vi "RTS Sequence Logic.vi"(4 "Relay Number":u8=1 min=1 max=3 step=1, 5 "Delay":bool, 6 "Current Status":string[](array[string]), 7 "Station 1-8 Data in":T2 {"Station Slide"."Chamber 1-1"."Start Time" format="%<%X\n%x>T"; "Station Slide"."Chamber 1-1"."End Time" format="%<%X\n%x>T"; "Station Slide"."Time Count (s)" format="%.2f"; "Station Cab"."Chamber 1-1"."Start Time" format="%<%X\n%x>T"; "Station Cab"."Chamber 1-1"."End Time" format="%<%X\n%x>T"; "Station Cab"."Time Count (s)" format="%.2f"; "Station Freezer"."Chamber 1-1"."Start Time" format="%<%X\n%x>T"; "Station Freezer"."Chamber 1-1"."End Time" format="%<%X\n%x>T"; "Station Freezer"."Time Count (s)" format="%.2f"}, 8 "error in (no error)":errorcluster, 10 "Door Open Delay(sec)":dbl, 11 "Door Open Sequence:":T1) -> (0 "error out":errorcluster, 2 "Run Door Op Sequence":bool, 3 "Station 1-8 Data out":T2 {"Station Slide"."Chamber 1-1"."Start Time" format="%<%X\n%x>T"; "Station Slide"."Chamber 1-1"."End Time" format="%<%X\n%x>T"; "Station Slide"."Time Count (s)" format="%.2f"; "Station Cab"."Chamber 1-1"."Start Time" format="%<%X\n%x>T"; "Station Cab"."Chamber 1-1"."End Time" format="%<%X\n%x>T"; "Station Cab"."Time Count (s)" format="%.2f"; "Station Freezer"."Chamber 1-1"."Start Time" format="%<%X\n%x>T"; "Station Freezer"."Chamber 1-1"."End Time" format="%<%X\n%x>T"; "Station Freezer"."Time Count (s)" format="%.2f"})   [LabVIEW 2016]
uses:
  Type Definitions/RTS Station Relay Ops.ctl
  Type Definitions/RTS Door Opener Indicator.ctl
  Type Definitions/RTS Door Ops Client.ctl
  Type Definitions/RTS Door Opening Schedule.ctl
  Type Definitions/RTS Door Ops Sequence.ctl
panel:
  # "Chamber Conditions:"
  # "Chamber Conditions:"
  # "Chamber Conditions:"
  # "Chamber Conditions:"
  # "Chamber Conditions:"
  # "Chamber Conditions:"
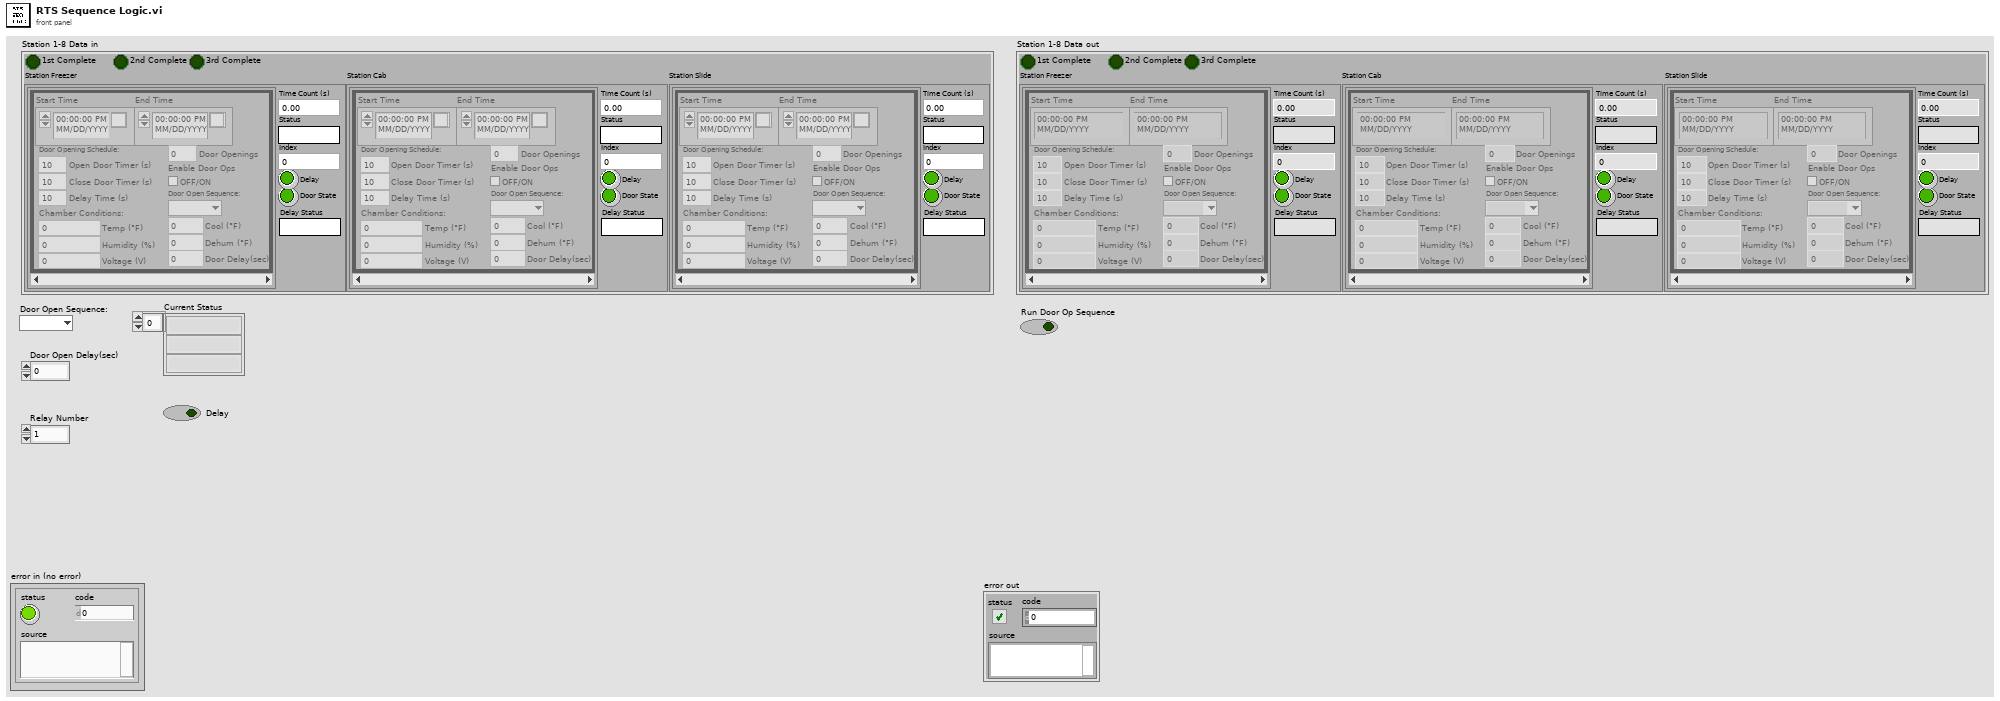
[diagram p1: front panel]
types:
  T1 = typedef "RTS Door Ops Sequence.ctl" = enum16{"", "1st", "2nd", "3rd"}
  T2 = typedef "RTS Station Relay Ops.ctl" = cluster{"Station Freezer":T3, "Station Cab":T3, "Station Slide":T3, "1st Complete":bool, "2nd Complete":bool, "3rd Complete":bool}
  T3 = typedef "RTS Door Opener Indicator.ctl" = cluster{"Time Count (s)":dbl, "Status":string, "Door State":bool, "Delay":bool, "Chamber 1-1":T4[], "Index":i32, "Delay Status":string}
  T4 = typedef "RTS Door Ops Client.ctl" = cluster{"End Time":timestamp, "Start Time":timestamp, "Door Opening Schedule:":T5, "Enable Door Ops":bool, "Door Openings":u32, "Temp (°F)":dbl, "Humidity (%)":dbl, "Voltage (V)":dbl, "Door Open Sequence:":T1, "Door Delay(sec)":dbl, "Dehum (°F)":dbl, "Cool (°F)":dbl}
  T5 = typedef "RTS Door Opening Schedule.ctl" = cluster{"Open Door Timer (s)":dbl, "Delay Time (s)":dbl, "Close Door Timer (s)":dbl}
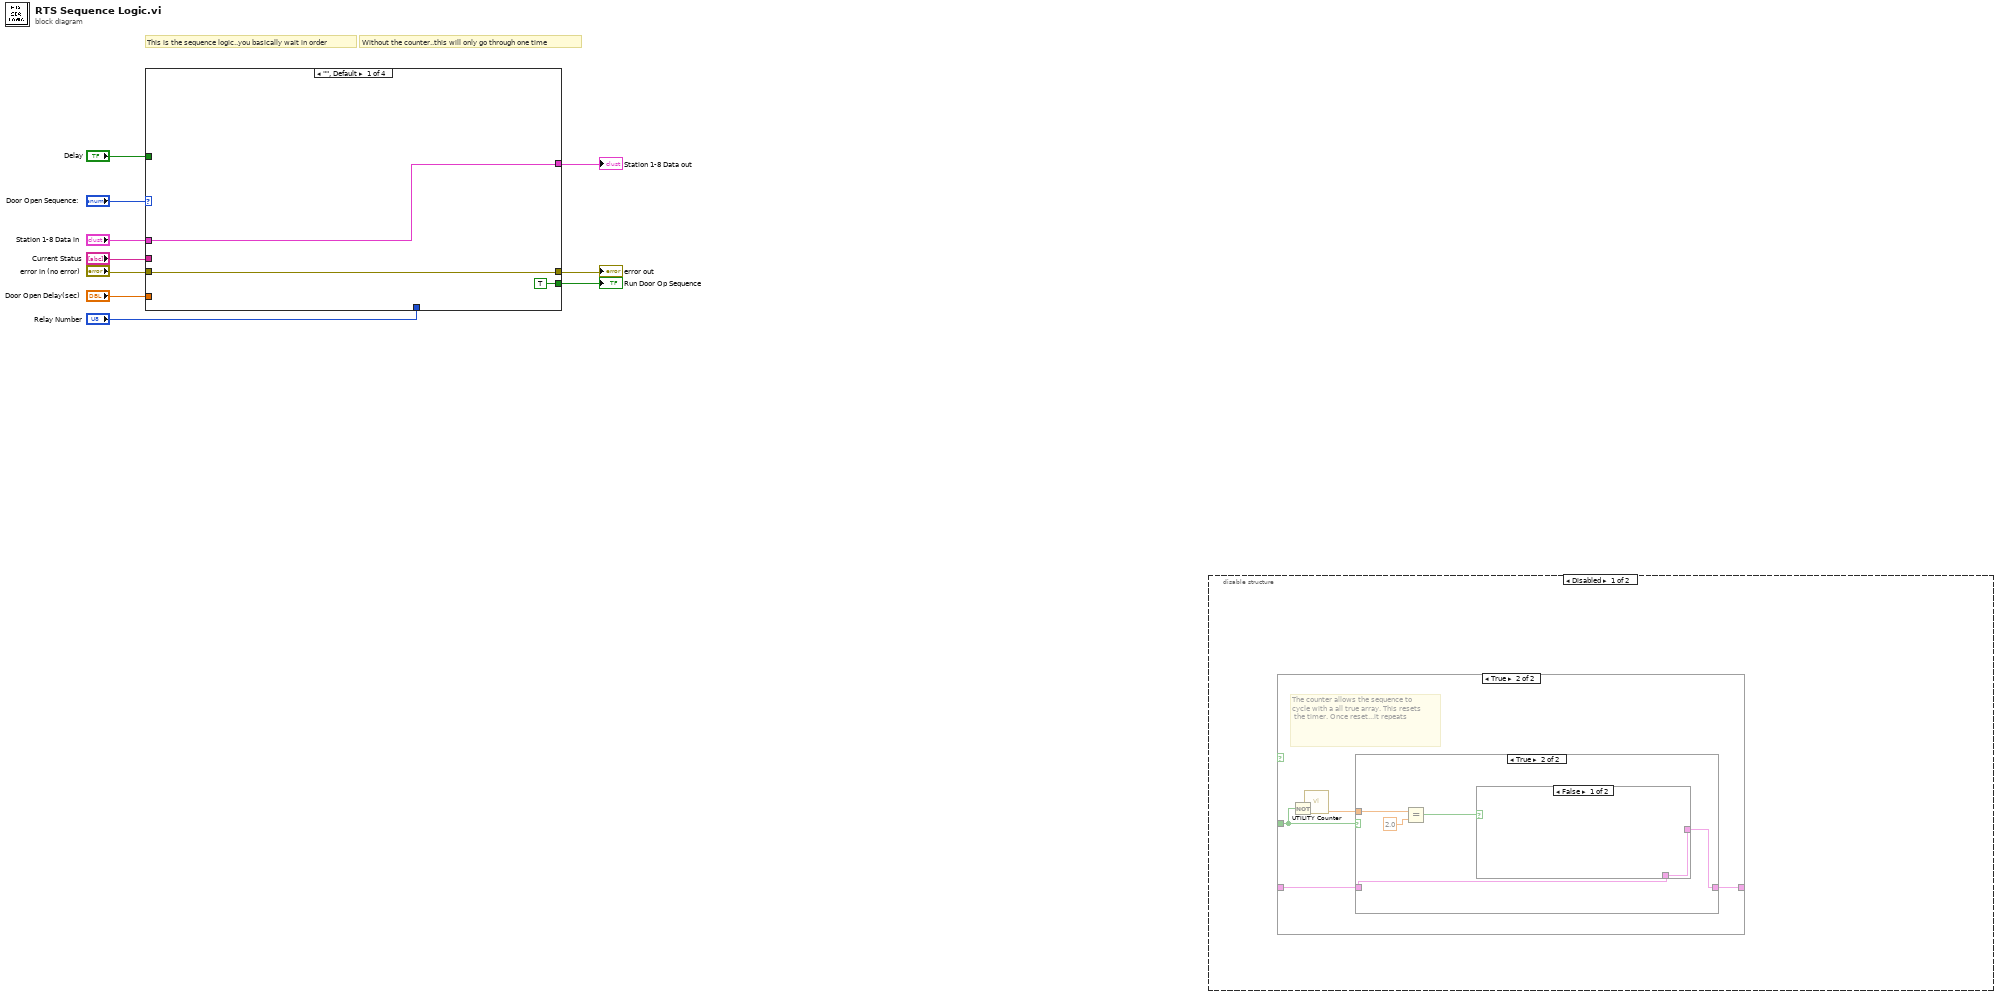
[diagram p0: block diagram]
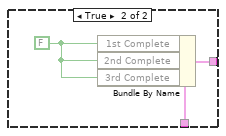
[diagram p4: hidden frame]
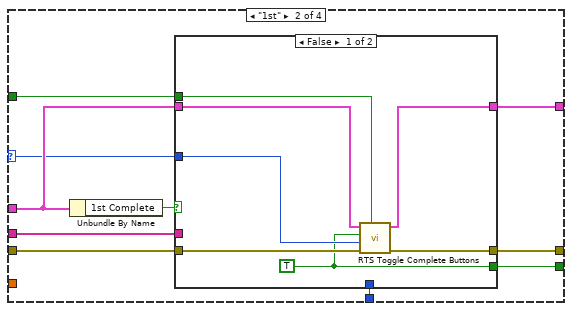
[diagram p6: hidden frame]
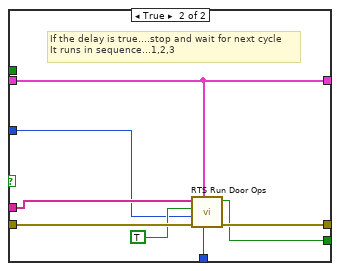
[diagram p7: hidden frame]
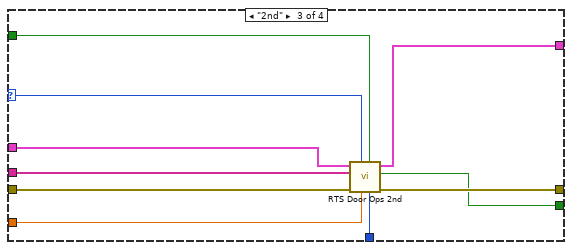
[diagram p8: hidden frame]
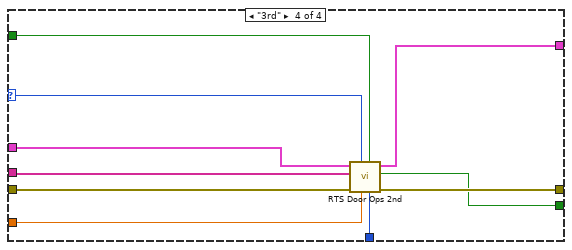
[diagram p9: hidden frame]
diagram:
  # "Without the counter..this will only go through one time"
  # "This is the sequence logic..you basically wait in order"
  n1 = case shown="\"\", Default" "Door Open Sequence:" {
    selector: "Door Open Sequence:" -> [_ w19 w41 w55]
    tunnel: "Door Open Delay(sec)" -> [_ _ w42 w56]
    tunnel: "error in (no error)" -> [w13 w18 w48 w58]
    tunnel: [w13 w17 w47 w57] -> w1
    tunnel: [TRUE ("Times Up?") w22 w46 w52] -> w3
    tunnel: "Station 1-8 Data in" -> [w11 w21 w44 w54]
    tunnel: [w11 w23 w45 w53] -> w2
    tunnel: "Current Status" -> [_ w16 w43 w51]
    tunnel: "Relay Number" -> [_ w15 w40 w50]
    tunnel: "Delay" -> [_ w14 w39 w49]
    frame "", Default {
    }
    frame "1st" {
      n2 = Unbundle By Name(w21) -> ("1st Complete"=w20:bool)
      n3 = case shown="False" w20 {
        tunnel: w21 -> [w30 w32]
        tunnel: [w29 w32] -> w23
        tunnel: [w25 w33] -> w22
        tunnel: w19 -> [w28 w34]
        tunnel: w18 -> [w27 w38]
        tunnel: [w26 w37] -> w17
        tunnel: w16 -> [_ w36]
        tunnel: w15 -> [_ w31]
        tunnel: w14 -> [w24 _]
        frame False {
          w25 = TRUE ("Times Up?")
          n4 = call "RTS Toggle Complete Buttons.vi"("Delay"=w24, "Error In"=w27, "Door Open Sequence:"=w28, "Times Up?"=w25, "Station 1-8 Data in in"=w30) -> ("Error Out"=w26:errorcluster, "Station 1-8 Data in out"=w29:T2)  [unwired: 5 in]
        }
        frame True {
          # "If the delay is true....stop and wait for next cycle\nIt runs in sequence...1,2,3"
          n5 = call "RTS Run Door Ops.vi"("Relay Number"=w31, "Station 1-8 Data in"=w32, "Error In"=w38, "Door Open Sequence:"=w34, "Complete?"=TRUE, "Current Status"=w36) -> ("Error Out"=w37:errorcluster, "Run Door Ops"=w33:bool)  [unwired: 3 in, 1 out]
        }
      }
    }
    frame "2nd" {
      n6 = call "RTS Door Ops 2nd.vi"("Relay Number"=w40, "Delay"=w39, "Door Open Delay(sec)"=w42, "Door Open Sequence:"=w41, "error in (no error)"=w48, "Current Status"=w43, "Station 1-8 Data in in"=w44) -> ("error out"=w47:errorcluster, "Run Door Ops"=w46:bool, "Station 1-8 Data out"=w45:T2)  [unwired: 1 in, 1 out]
    }
    frame "3rd" {
      n7 = call "RTS Door Ops 2nd.vi"("Relay Number"=w50, "Delay"=w49, "Door Open Delay(sec)"=w56, "Door Open Sequence:"=w55, "error in (no error)"=w58, "Current Status"=w51, "Station 1-8 Data in in"=w54) -> ("error out"=w57:errorcluster, "Run Door Ops"=w52:bool, "Station 1-8 Data out"=w53:T2)  [unwired: 1 in, 1 out]
    }
  }
  "Station 1-8 Data out" <- w2
  "error out" <- w1
  "Run Door Op Sequence" <- w3
  n8 = disable-structure shown="Disabled" {
    frame Disabled {
      n9 = case shown="True" {
        selector: _ -> [_ _]
        tunnel: _ -> [w59 w64]
        tunnel: [w59 w63] -> _
        tunnel: _ -> [_ w62]
        frame False {
        }
        frame True {
          # "The counter allows the sequence to\ncycle with a all true array. This resets\n the timer. Once reset...it repeats"
          n10 = Not(x=w62) -> (.not. x?=w61:bool)
          n11 = call "UTILITY Counter.vi"("Reset"=w61) -> ("Count"=w60:dbl)  [unwired: 10 in]
          n12 = case shown="True" w62 {
            tunnel: w64 -> [w65 w67]
            tunnel: [w65 w66] -> w63
            tunnel: w60 -> [_ w70]
            frame False {
            }
            frame True {
              n13 = Equal?(x=w70, y=2.0) -> (x = y?=w68:bool)
              n14 = case shown="False" w68 {
                tunnel: w67 -> [w71 w74]
                tunnel: [w71 w73] -> w66
                frame False {
                }
                frame True {
                  w72 = FALSE ("1st Complete")
                  n15 = Bundle By Name(cluster=w74, "1st Complete"=w72, "2nd Complete"=w72, "3rd Complete"=w72) -> (w73:cluster{})
                }
              }
            }
          }
        }
      }
    }
    frame Enabled {
    }
  }
